vi "Generate Sample Channel Data.vi"(9 "channel type":T1 items=["Pulsing Sine Wave", "Fixed Sine Wave", "Drifting Sine Wave"], 10 "channel idx":i32, 11 "sample size":i32) -> (3 "channel data":csg[](array[numeric]))   [LabVIEW 2020, in "Multi-channel FFT.lvlib"]
uses:
  Multi-channel FFT.lvlib
  Channel Data Type.ctl
  <vilib>/Analysis/NI_AALBase.lvlib
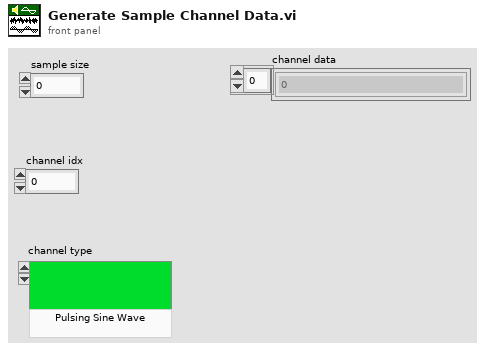
[diagram p1: front panel]
types:
  T1 = typedef "Multi-channel FFT.lvlib/Channel Data Type.ctl" = u16
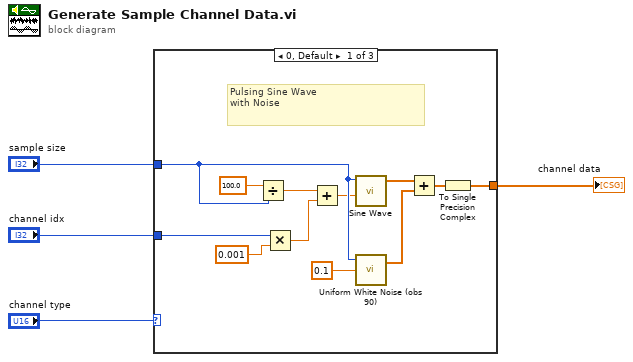
[diagram p0: block diagram]
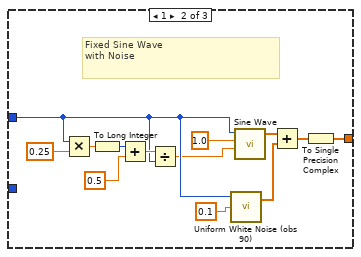
[diagram p2: hidden frame]
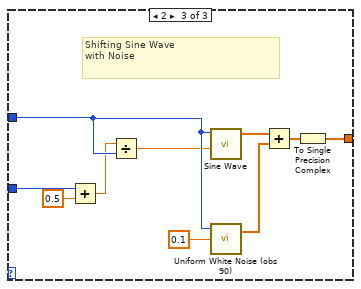
[diagram p3: hidden frame]
diagram:
  n1 = case shown="0, Default" "channel type" {
    tunnel: "sample size" -> [w16 w18 w34]
    tunnel: [w8 w26 w36] -> w3
    tunnel: "channel idx" -> [w6 _ w31]
    frame 0, Default {
      # "Pulsing Sine Wave\nwith Noise"
      n2 = Divide(x=100.0 ("Cursor.Cursor Position:Cursor Y"), y=w16) -> (x/y=w9:dbl)
      n3 = Multiply(x=w6, y=0.001) -> (x*y=w15:dbl)
      n4 = Add(x=w9, y=w15) -> (x+y=w10:dbl)
      n5 = call <vilib>:"Sine Wave.vi"("samples"=w16, "frequency"=w10) -> ("sine wave"=w11:dbl[])  [unwired: 3 in, 2 out]
      n6 = call <vilib>:"Uniform White Noise (obs 90).vi"("amplitude"=0.1 ("standard deviation"), "samples"=w16) -> ("uniform white noise"=w12:dbl[])  [unwired: 1 in, 1 out]
      n7 = Add(x=w11, y=w12) -> (x+y=w7:dbl[])
      n8 = To Single Precision Complex(1:w7) -> (0:w8:csg[])
    }
    frame 1 {
      # "Fixed Sine Wave\nwith Noise"
      n9 = Multiply(x=w18, y=0.25 ("frequency")) -> (x*y=w22:dbl)
      n10 = To Long Integer(number=w22) -> (32bit integer=w20:i32)
      n11 = Add(x=w20, y=0.5) -> (x+y=w19:dbl)
      n12 = Divide(x=w19, y=w18) -> (x/y=w17:dbl)
      n13 = call <vilib>:"Uniform White Noise (obs 90).vi"("amplitude"=0.1 ("standard deviation"), "samples"=w18) -> ("uniform white noise"=w28:dbl[])  [unwired: 1 in, 1 out]
      n14 = call <vilib>:"Sine Wave.vi"("samples"=w18, "amplitude"=1.0, "frequency"=w17) -> ("sine wave"=w27:dbl[])  [unwired: 2 in, 2 out]
      n15 = Add(x=w27, y=w28) -> (x+y=w25:dbl[])
      n16 = To Single Precision Complex(1:w25) -> (0:w26:csg[])
    }
    frame 2 {
      # "Shifting Sine Wave\nwith Noise"
      n17 = Add(x=w31, y=0.5) -> (x+y=w32:dbl)
      n18 = Divide(x=w32, y=w34) -> (x/y=w33:dbl)
      n19 = call <vilib>:"Sine Wave.vi"("samples"=w34, "frequency"=w33) -> ("sine wave"=w37:dbl[])  [unwired: 3 in, 2 out]
      n20 = call <vilib>:"Uniform White Noise (obs 90).vi"("amplitude"=0.1 ("standard deviation"), "samples"=w34) -> ("uniform white noise"=w38:dbl[])  [unwired: 1 in, 1 out]
      n21 = Add(x=w37, y=w38) -> (x+y=w35:dbl[])
      n22 = To Single Precision Complex(1:w35) -> (0:w36:csg[])
    }
  }
  "channel data" <- w3
